vi "Helmholtz2D_FEM_Check Input_BC.vi"(8 "error in (no error)":errorcluster, 10 "Domain":cluster{"X":dbl[], "Y":dbl[]}, 11 "Boundary Condition":cluster{"type":T1, "Value":dbl[]} {"type" items=["Dirichlet", "Neumann"]}) -> (0 "error out":errorcluster)   [LabVIEW 2017, in "NI_PDE.lvlib"]
uses:
  <vilib>/gmath/NI_PDE.lvlib
  <vilib>/gmath/pde.llb/Common/PDE_BC Type.ctl
  <vilib>/gmath/pde.llb/Common/PDE_Error.ctl
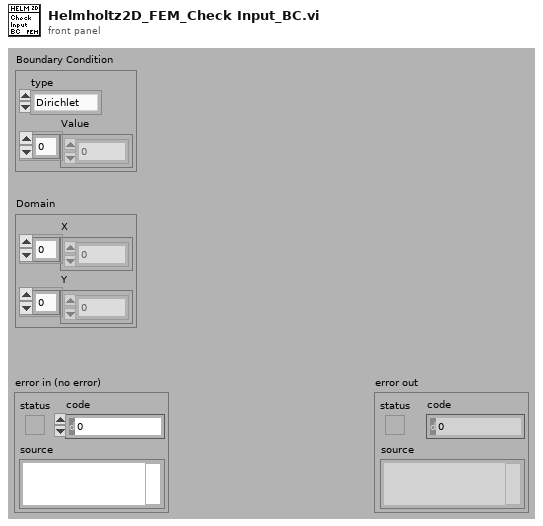
[diagram p1: front panel]
types:
  T1 = typedef "NI_PDE.lvlib/PDE_BC Type.ctl" = i32
  T2 = typedef "NI_PDE.lvlib/PDE_Error.ctl" = enum16{"No Error", "k is zero", "End point <= start point", "# of time steps < 2", "# of spatial points < 3", "# of grid < 1 for FEM", "# of boundary < 3 for FEM", "Incompatible RHS size", "Incompatible BC size", "Incompatible IC size", "PDE class conflict", "RHS class conflict", "Domain class conflict", "BC class conflict", "IC class conflict"}
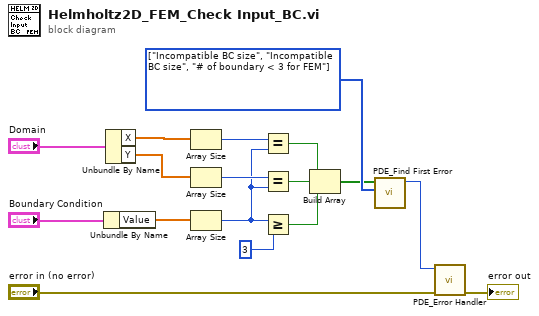
[diagram p0: block diagram]
diagram:
  w13 = T2[] [enum."Incompatible BC size", enum."Incompatible BC size", enum."# of boundary < 3 for FEM"] items=["No Error", "k is zero", "End point <= start point", "# of time steps < 2", "# of spatial points < 3", "# of grid < 1 for FEM", "# of boundary < 3 for FEM", "Incompatible RHS size", "Incompatible BC size", "Incompatible IC size", "PDE class conflict", "RHS class conflict", "Domain class conflict", "BC class conflict", "IC class conflict"]
  n1 = Unbundle By Name("Boundary Condition") -> ("Value"=w4:dbl[])
  n2 = Unbundle By Name("Domain") -> ("X"=w6:dbl[], "Y"=w5:dbl[])
  n3 = Array Size(array=w6) -> (size(s)=w12:i32)
  n4 = Array Size(array=w5) -> (size(s)=w11:i32)
  n5 = Array Size(array=w4) -> (size(s)=w3:i32)
  n6 = Equal?(x=w12, y=w3) -> (x = y?=w10:bool)
  n7 = Equal?(x=w11, y=w3) -> (x = y?=w9:bool)
  n8 = Greater Or Equal?(x=w3, y=3 ("x")) -> (x >= y?=w2:bool)
  n9 = Build Array(w10, w9, w2) -> (w8:bool[])
  n10 = call <vilib>:"PDE_Find First Error.vi"("PDE Error"=w13, "Failure"=w8) -> ("first error"=w14:T2)  [unwired: 9 out]
  n11 = call <vilib>:"PDE_Error Handler.vi"("error in (no error)"="error in (no error)", "PDE error"=w14) -> ("error out"=→"error out":errorcluster)  [unwired: 9 out]
